vi "ToTable Test.vi"() -> (0 "error out":errorcluster)   [LabVIEW 2015, in "E2E Tag Exchange tests.lvlib"]
doc: "Tests the 'To Table' method."
uses:
  E2E Tag Exchange tests.lvlib
  <vilib>/NI/Module Execution Interface/Engine Configuration/engine configuration.lvclass
  editor node/E2E Tag Exchange editor node.lvclass
  <vilib>/NI/Configuration Framework/serializable configuration/NISE_CEF_serializable configuration.lvclass/NISE_CEF_serializable configuration.ctl
  <vilib>/Utility/LVClass/Get LV Class Name.vi
  <vilib>/NI/Configuration Framework/error generator/NISE_error generator.vi
  <vilib>/NI/Configuration Framework/serializable configuration/NISE_CEF_serializable configuration.lvclass
panel:
  out "table":string[][](array[string])
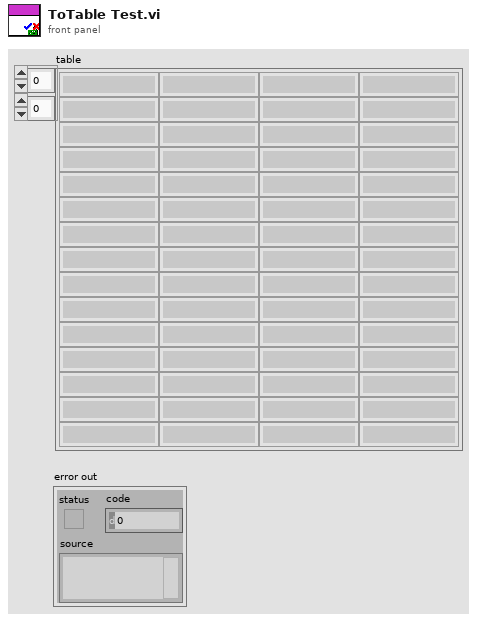
[diagram p1: front panel]
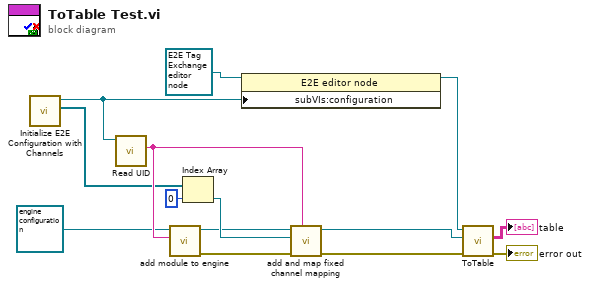
[diagram p0: block diagram]
diagram:
  n1 = call "Initialize E2E Configuration with Channels.vi"() -> ("Random Channels Added"=w2:refnum<class "TBM channel.lvclass">[], "Initialized E2E configuration"=w3:refnum<class "E2E Tag Exchange configuration.lvclass">)  [unwired: 9 in, 1 out]
  n2 = call <vilib>:"Read UID.vi"("configuration in"=w3) -> ("instance id"=w6:string)  [unwired: 8 in, 2 out]
  n3 = call-dynamic "add module to engine.vi"("module ID"=w6, "engine configuration in"=refnum<class "engine configuration.lvclass"> refnum ("engine configuration")) -> ("error out"=w5:errorcluster, "engine configuration out"=w7:refnum<class "engine configuration.lvclass">)  [unwired: 8 in]
  n4 = Index Array(array=w2, index=0) -> (element=w9:refnum<class "TBM channel.lvclass">)
  n5 = property class="E2E editor node"(reference=refnum<class "E2E Tag Exchange editor node.lvclass"> refnum ("node in"), "subVIs:configuration"=w3) -> (reference out=w13:refnum<class "E2E Tag Exchange editor node.lvclass">)  [unwired: 1 in, 1 out]
  n6 = call <vilib>:"add and map fixed channel mapping.vi"("module instance"=w6, "error in"=w5, "fixed channel"=w9, "engine configuration in"=w7) -> ("error out"=w4:errorcluster, "engine configuration out"=w8:refnum<class "engine configuration.lvclass">)  [unwired: 6 in]
  n7 = call-dynamic "ToTable.vi"("error in (no error)"=w4, "variant"=w8, "node in"=w13) -> ("error out"=→"error out":errorcluster, "table"=→"table":string[][])  [unwired: 5 in, 2 out]
